vi "_TO BE DELETED Populate SCLs.vi"(8 "error in":errorcluster, 11 "SCL":refnum<vi>) -> (0 "error out":errorcluster, 3 "Section Header Indexes":i32[](array[numeric]))   [LabVIEW 2020]
doc: "Populates the two SCLs that display the available VI templates and CTL templates, respectively.\n\nSCL = Single-Column Listbox"
uses:
  <vilib>/Utility/miscctls.llb/LVFontTypeDef.ctl
panel:
  out "VIs":string[](array[string])
  out "CTLs":string[](array[string])
  out "Templates Folder Location":path
  out "All Filenames":string[](array[string])
  # "Development\ncontrols/indicators useful for development and testing, but which are not outputs of the VI"
  # "Input\nInputs to the VI"
  # "Output\nOutputs of the VI"
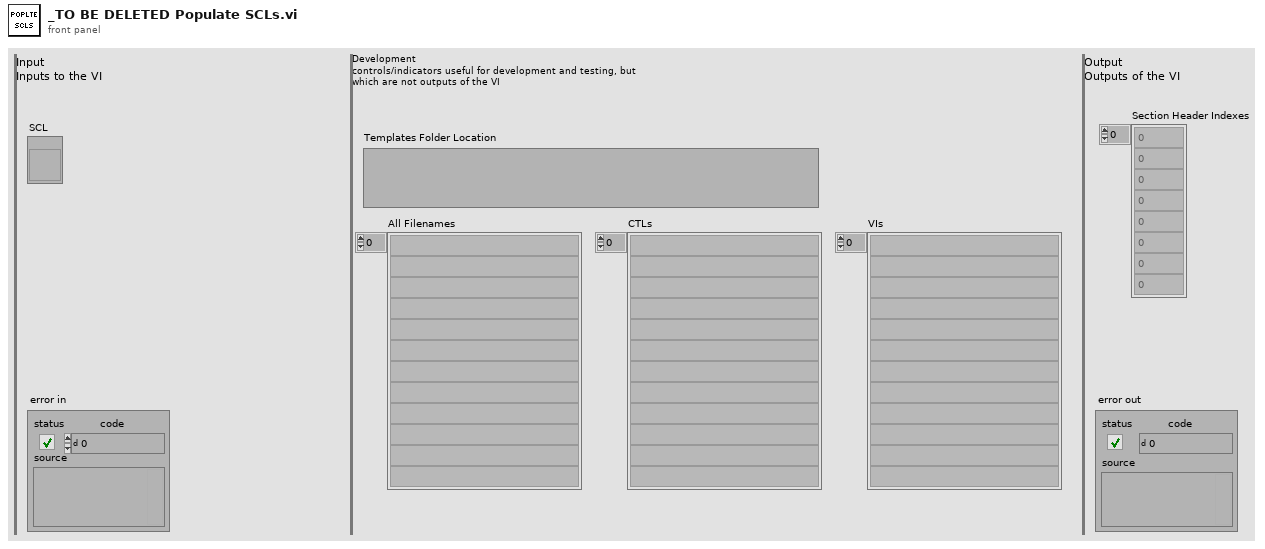
[diagram p1: front panel]
types:
  T1 = typedef "LVFontTypeDef.ctl" = cluster{"Font Name":string, "Size":u16, "Bold":bool, "Italic":bool, "Underline":bool, "Strikeout":bool, "Color":u32}
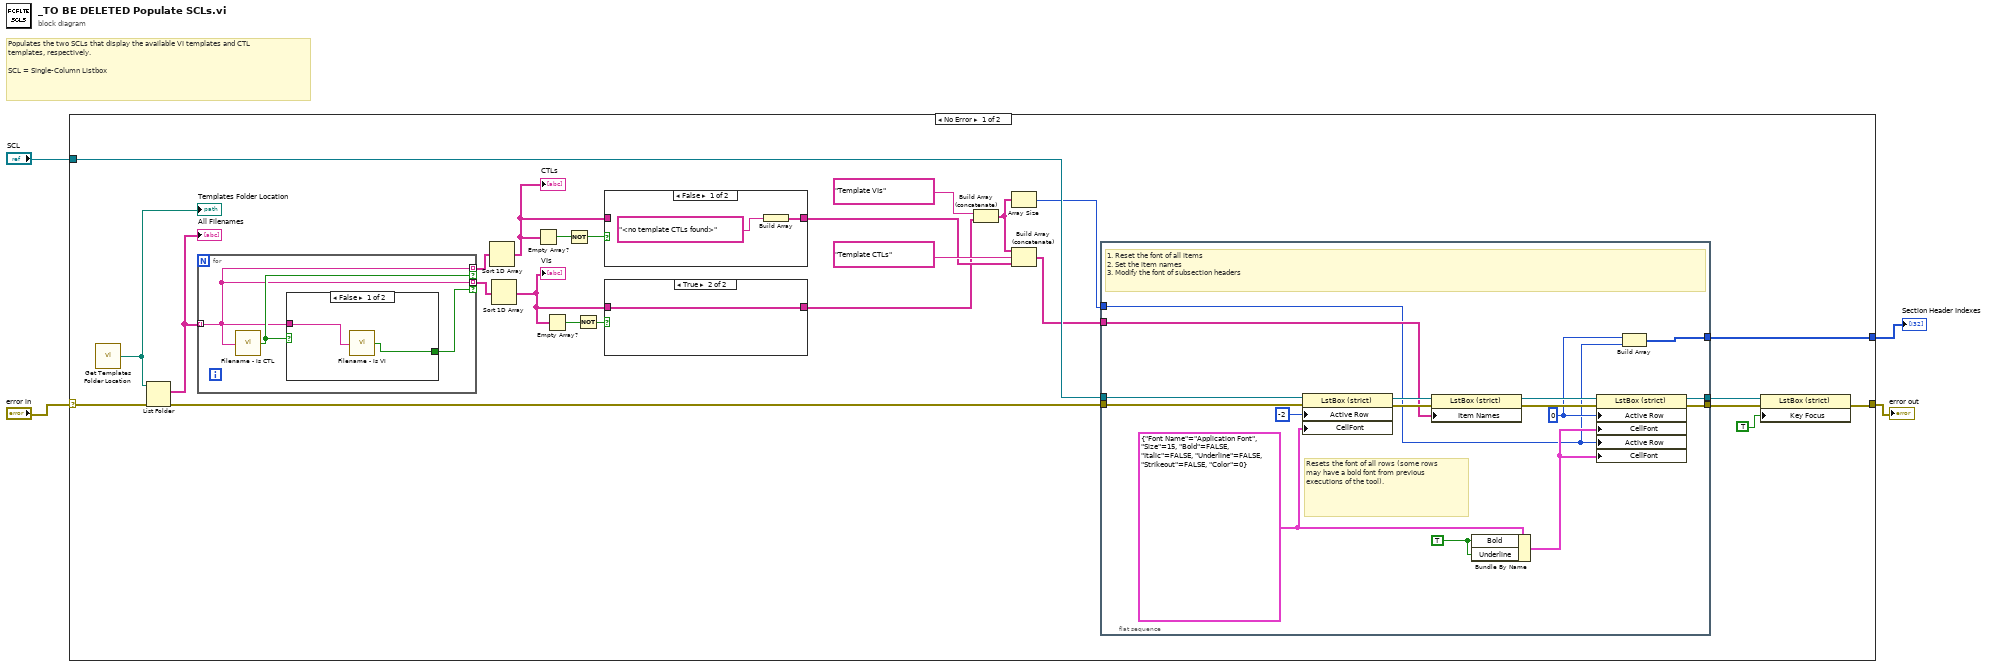
[diagram p0: block diagram]
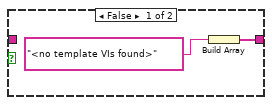
[diagram p3: hidden frame]
diagram:
  # "Populates the two SCLs that display the available VI templates and CTL templates, respectively.\n\nSCL = Single-Column Listbox"
  n1 = case shown="No Error" "error in" {
    selector: "error in" -> [w29 w57]
    tunnel: [w8 w57] -> w3
    tunnel: "SCL" -> [w24 _]
    tunnel: [w5 _] -> w1
    frame No Error {
      n2 = call "Get Templates Folder Location.vi"() -> ("Templates Folder Location"=w9:path)
      "Templates Folder Location" <- w9
      n3 = List Folder(path=w9, error in=w29) -> (filenames=w27:string[], error out=w28:errorcluster)  [unwired: 2 in, 2 out]
      "All Filenames" <- w27
      n4 = for {
        tunnel: w27 -> [w46] mode=indexing
        tunnel: [w46] -> w26 mode=indexing if=w47
        tunnel: [w46] -> w25 mode=indexing if=w48
        n5 = call "Filename - Is CTL.vi"("Filename (including file extension)"=w46) -> ("Is CTL?"=w47:bool)
        n6 = case shown="False" w47 {
          tunnel: [w49 _] -> w48
          tunnel: w46 -> [w50 _]
          frame False {
            n7 = call "Filename - Is VI.vi"("Filename (including file extension)"=w50) -> ("Is VI?"=w49:bool)
          }
          frame True {
          }
        }
      }
      n8 = Sort 1D Array(array=w26) -> (sorted array=w21:string[])
      "CTLs" <- w21
      n9 = Sort 1D Array(array=w25) -> (sorted array=w19:string[])
      "VIs" <- w19
      n10 = Empty Array?(array=w21) -> (empty?=w23:bool)
      n11 = Empty Array?(array=w19) -> (empty?=w20:bool)
      n12 = Not(x=w23) -> (.not. x?=w22:bool)
      n13 = Not(x=w20) -> (.not. x?=w18:bool)
      n14 = case shown="False" w22 {
        tunnel: w21 -> [_ w56]
        tunnel: [w54 w56] -> w14
        frame False {
          n15 = Build Array("<no template CTLs found>") -> (w54:string[])
        }
        frame True {
        }
      }
      n16 = case shown="True" w18 {
        tunnel: w19 -> [_ w53]
        tunnel: [w51 w53] -> w13
        frame False {
          n17 = Build Array("<no template VIs found>") -> (w51:string[])
        }
        frame True {
        }
      }
      n18 = Build Array (concatenate)("Template VIs", w13) -> (w16:string[])
      n19 = Array Size(array=w16) -> (size(s)=w11:i32)
      n20 = Build Array (concatenate)(w16, "Template CTLs", w14) -> (w12:string[])
      n21 = flat-sequence {
        tunnel: w28 -> [w45]
        tunnel: w24 -> [w44]
        tunnel: w12 -> [w40]
        tunnel: w11 -> [w30]
        tunnel: [w35] -> w10
        tunnel: [w33] -> w7
        tunnel: [w31] -> w5
        frame #0 {
          w34 = TRUE ("Bold")
          w32 = 0 ("Active Row:Active Row Number")
          w37 = T1 {"Font Name"="Application Font", "Size"=15, "Bold"=FALSE, "Italic"=FALSE, "Underline"=FALSE, "Strikeout"=FALSE, "Color"=0} ("Active Row:Cell Font")
          # "Resets the font of all rows (some rows may have a bold font from previous executions of the tool)."
          # "1. Reset the font of all items\n2. Set the item names\n3. Modify the font of subsection headers"
          n22 = property class="LstBox (strict)"(reference=w44, error in=w45, "Active Row"=-2 ("Active Row:Active Row Number"), "CellFont"=w37) -> (reference out=w42:refnum<vi>, error out=w41:errorcluster)
          n23 = property class="LstBox (strict)"(reference=w42, error in=w41, "Item Names"=w40) -> (reference out=w38:refnum<vi>, error out=w39:errorcluster)
          n24 = Bundle By Name(cluster=w37, "Bold"=w34, "Underline"=w34) -> (w36:T1)
          n25 = property class="LstBox (strict)"(reference=w38, error in=w39, "Active Row"=w32, "CellFont"=w36, "Active Row"=w30, "CellFont"=w36) -> (reference out=w33:refnum<vi>, error out=w35:errorcluster)
          n26 = Build Array(w32, w30) -> (w31:i32[])
        }
      }
      n27 = property class="LstBox (strict)"(reference=w7, error in=w10, "Key Focus"=TRUE) -> (error out=w8:errorcluster)  [unwired: 1 out]
    }
    frame Error {
    }
  }
  "error out" <- w3
  "Section Header Indexes" <- w1
